vi "Keithley 6517A LTCC Single Read2.vi"(8 "error in":T1, 9 "Read Displays":bool=TRUE, 10 "Scanner Channel":i16=1 min=1 max=10 step=1, 11 "GPIB address":string="27") -> (0 "error out":T1, 1 "time and date stamp":string, 2 "Time":string, 3 "measurement":dbl=-0.0 format="%.6e", 4 "secondary display":string="\n", 5 "units":string="0", 6 "reading #":dbl, 7 "primary display":string="\n")   [LabVIEW 2013]
doc: "This VI takes a single reading from the 6517. The data returned includes the reading, timestamp, units, and reading#."
panel:
  in  "poll enable":bool
  in  "Zero Check":bool=TRUE
  out "Raw Readback":string="\n"
  # "(A)"
  # "ON\nOFF"
  # "ON\nOFF"
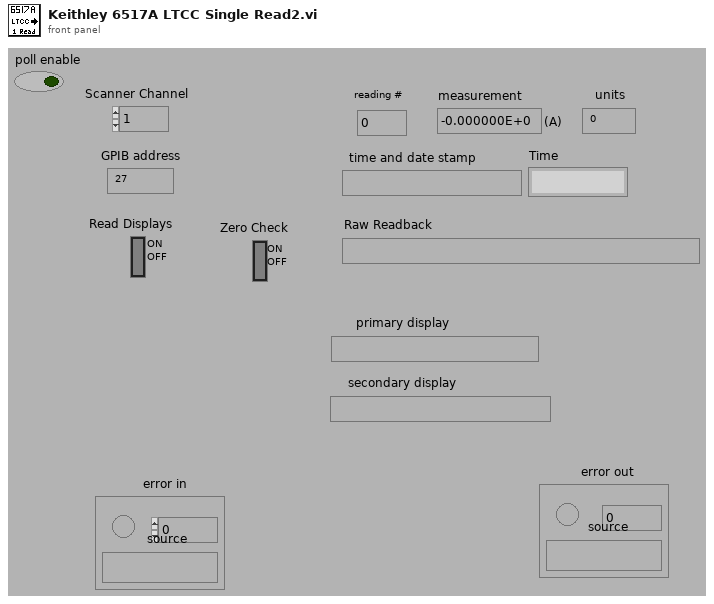
[diagram p1: front panel]
types:
  T1 = cluster{"error":bool, "code":i32, "source":string}
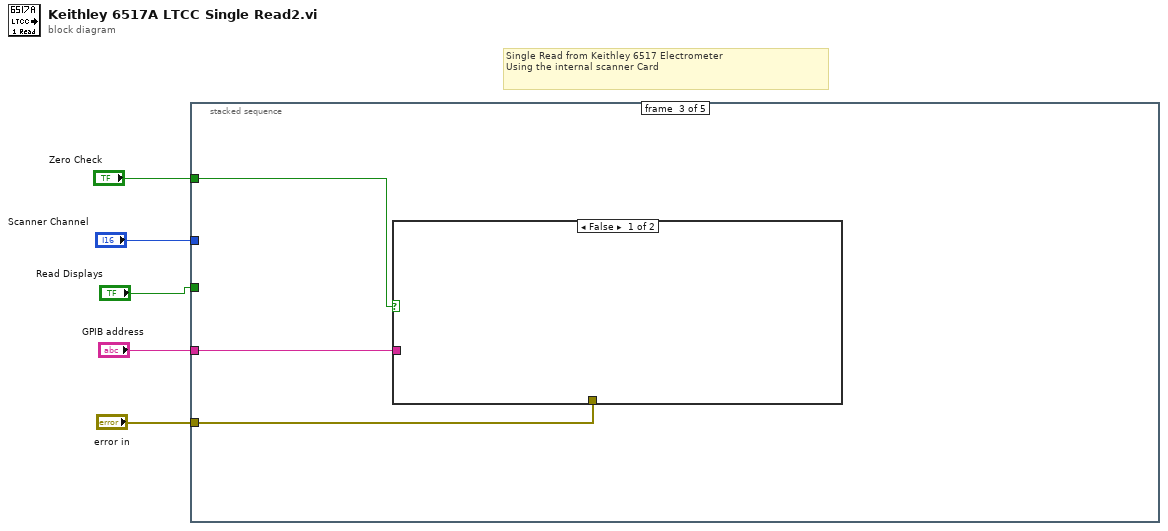
[diagram p0: block diagram]
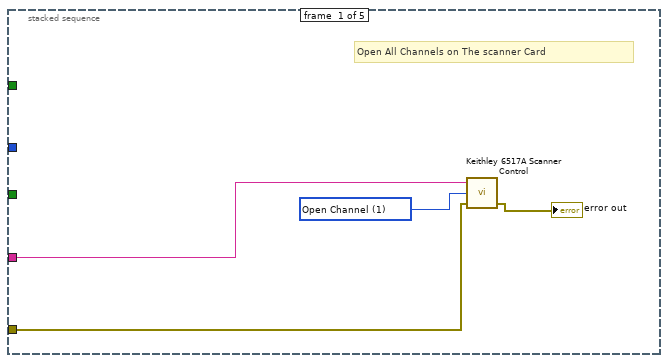
[diagram p2: hidden frame]
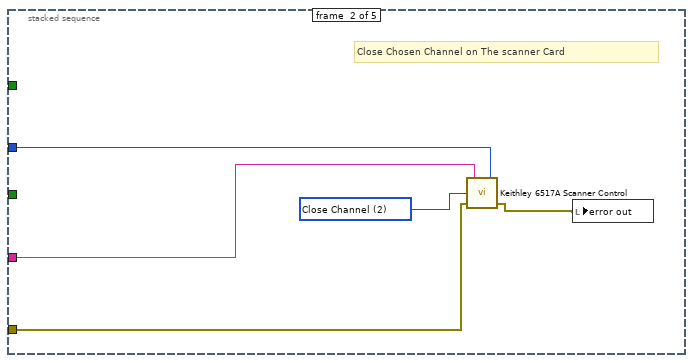
[diagram p3: hidden frame]
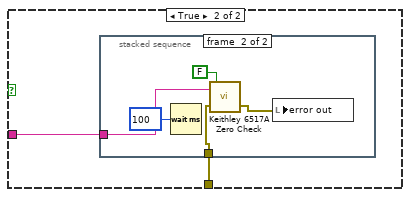
[diagram p4: hidden frame]
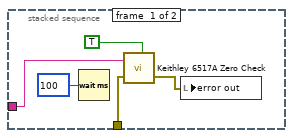
[diagram p5: hidden frame]
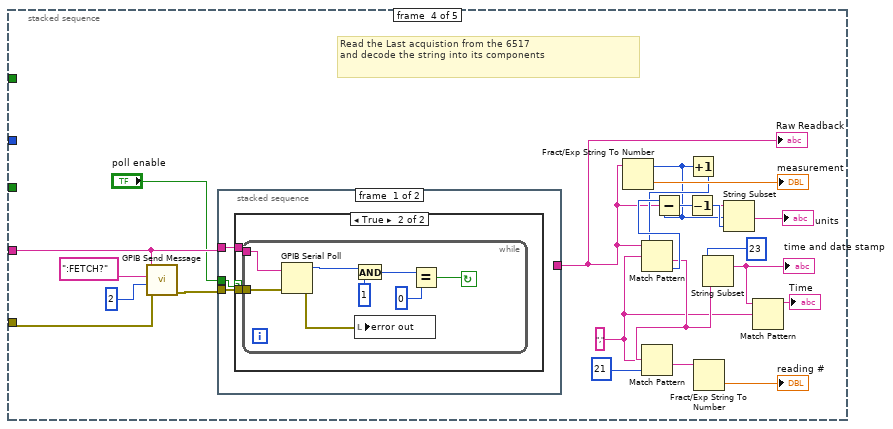
[diagram p6: hidden frame]
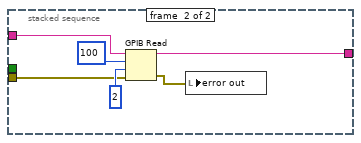
[diagram p8: hidden frame]
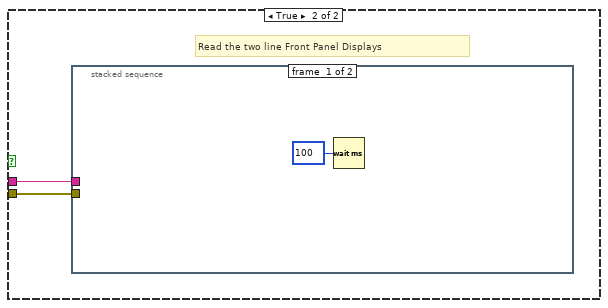
[diagram p10: hidden frame]
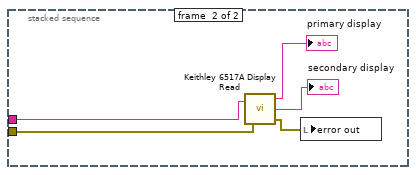
[diagram p11: hidden frame]
diagram:
  # "Single Read from Keithley 6517 Electrometer \nUsing the internal scanner Card"
  n1 = stacked-sequence {
    tunnel: "GPIB address" -> [w6 w12 w15 w36 w72]
    tunnel: "error in" -> [w9 w14 w16 w34 w71]
    tunnel: "Scanner Channel" -> [_ w10 _ _ _]
    tunnel: "Read Displays" -> [_ _ _ _ w73]
    tunnel: "Zero Check" -> [_ _ w17 _ _]
    frame #0 {
      w8 = u16 1 items=["Open All", "Open Channel", "Close Channel", "Scan List"] ("Scanner Control")
      # "Open All Channels on The scanner Card"
      n2 = call "Keithley 6517A Scanner Control.vi"("error in"=w9, "Scanner Control"=w8, "GPIB address"=w6) -> ("error out"=→"error out":T1)  [unwired: 2 in]
    }
    frame #1 {
      w13 = u16 2 items=["Open All", "Open Channel", "Close Channel", "Scan List"] ("Scanner Control")
      # "Close Chosen Channel on The scanner Card"
      n3 = call "Keithley 6517A Scanner Control.vi"("Open / Close Internal Scanner Channel"=w10, "error in"=w14, "Scanner Control"=w13, "GPIB address"=w12) -> ("error out"=w11:T1)  [unwired: 1 in]
      n4 = local write "error out"(w11) -> ()
    }
    frame #2 {
      n5 = case shown="False" w17 {
        tunnel: w16 -> [_ w19]
        tunnel: w15 -> [_ w18]
        frame False {
        }
        frame True {
          n6 = stacked-sequence {
            tunnel: w19 -> [w24 w29]
            tunnel: w18 -> [w23 w28]
            frame #0 {
              n7 = Wait (ms)(milliseconds to wait=u32 100) -> ()  [unwired: 1 out]
              n8 = call "Keithley 6517A Zero Check.vi"("Zero Check"=TRUE, "error in"=w24, "GPIB address"=w23) -> ("error out"=w21:T1)
              n9 = local write "error out"(w21) -> ()
            }
            frame #1 {
              n10 = Wait (ms)(milliseconds to wait=u32 100) -> ()  [unwired: 1 out]
              n11 = call "Keithley 6517A Zero Check.vi"("Zero Check"=FALSE, "error in"=w29, "GPIB address"=w28) -> ("error out"=w26:T1)
              n12 = local write "error out"(w26) -> ()
            }
          }
        }
      }
    }
    frame #3 {
      w33 = ","
      # "Read the Last acquistion from the 6517\nand decode the string into its components"
      n13 = call "GPIB Send Message.vi"("address string"=w36, "write buffer"=":FETCH?", "write mode (set END:0)"=2, "error in"=w34) -> ("error out"=w37:T1)  [unwired: 3 in, 2 out]
      n14 = stacked-sequence {
        tunnel: [_ w70] -> w35
        tunnel: w37 -> [w53 w67]
        tunnel: w36 -> [w54 w66]
        tunnel: "poll enable" -> [w52 _]
        frame #0 {
          n15 = case shown="True" w52 {
            tunnel: w54 -> [_ w56]
            tunnel: w53 -> [_ w55]
            frame False {
            }
            frame True {
              n16 = while {
                tunnel: w56 -> [w59]
                tunnel: w55 -> [w58]
                stop <- w63 continue-if-true
                n17 = GPIB Serial Poll(0:w59, 1:w58) -> (2:w62:i16, 4:w57:errorcluster)  [unwired: 1 out]
                n18 = And(x=w62, y=1) -> (x .and. y?=w60:i32)
                n19 = local write "error out"(w57) -> ()
                n20 = Equal?(x=w60, y=0) -> (x = y?=w63:bool)
              }
            }
          }
        }
        frame #1 {
          n21 = GPIB Read(0:w66, 1:100, 2:2, 3:w67) -> (5:w70:string, 7:w65:errorcluster)  [unwired: 1 in, 1 out]
          n22 = local write "error out"(w65) -> ()
        }
      }
      "Raw Readback" <- w35
      n23 = Fract/Exp String To Number(string=w35) -> (offset past number=w40:i32, number=→"measurement":dbl)  [unwired: 3 in]
      n24 = Increment(x=w40) -> (x+1=w41:i32)
      n25 = Match Pattern(string=w35, regular expression=w33, offset (0)=w41) -> (after substring=w43:string, offset past match=w47:i32)  [unwired: 2 out]
      n26 = Match Pattern(string=w43, regular expression=w33, offset (0)=21) -> (after substring=w48:string)  [unwired: 3 out]
      n27 = Subtract(x=w47, y=w40) -> (x-y=w45:i32)
      n28 = Decrement(x=w45) -> (x-1=w46:i32)
      n29 = Fract/Exp String To Number(string=w48) -> (number=→"reading #":dbl)  [unwired: 3 in, 1 out]
      n30 = String Subset(string=w43, length (rest)=23) -> (substring=w32:string)  [unwired: 1 in]
      "time and date stamp" <- w32
      n31 = String Subset(string=w35, offset (0)=w40, length (rest)=w46) -> (substring=→"units":string)
      n32 = Match Pattern(string=w32, regular expression=w33) -> (before substring=→"Time":string)  [unwired: 1 in, 3 out]
    }
    frame #4 {
      n33 = case shown="False" w73 {
        tunnel: w72 -> [_ w75]
        tunnel: w71 -> [_ w74]
        frame False {
        }
        frame True {
          # "Read the two line Front Panel Displays"
          n34 = stacked-sequence {
            tunnel: w75 -> [_ w81]
            tunnel: w74 -> [_ w80]
            frame #0 {
              n35 = Wait (ms)(milliseconds to wait=u32 100) -> ()  [unwired: 1 out]
            }
            frame #1 {
              n36 = call "Keithley 6517A Display Read.vi"("GPIB address"=w81, "error in"=w80) -> ("primary display"=→"primary display":string, "secondary display"=→"secondary display":string, "error out"=w77:T1)
              n37 = local write "error out"(w77) -> ()
            }
          }
        }
      }
    }
  }
